vi "Neocera21 Set T.vi"(5 "Channel":i16=1, 6 "Ramp rate, K/min":dbl=1.0, 8 "error in (no error)":errorcluster, 9 "Approach":T1, 10 "Set T":dbl=1.0, 11 "VISA Resource Name":refnum<visa-resource-name>) -> (0 "error out":errorcluster, 3 "VISA Resource Name Out":refnum<visa-resource-name>)   [LabVIEW 2021]
uses:
  Temperature Controller/Controls/Set Point Aproach.ctl
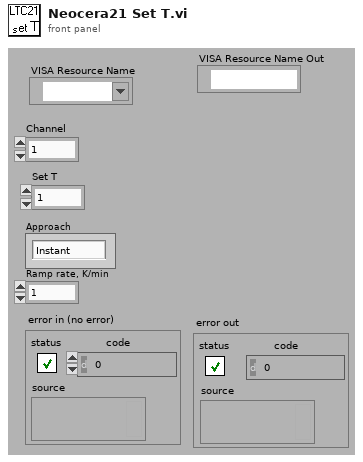
[diagram p1: front panel]
types:
  T1 = typedef "Set Point Aproach.ctl" = enum16{"Instant", "Ramp"}
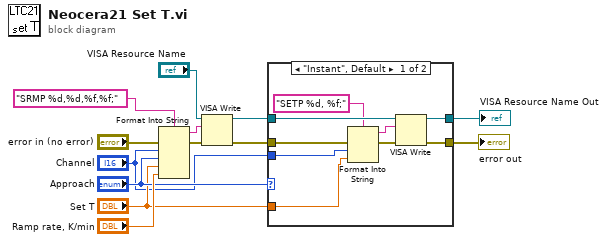
[diagram p0: block diagram]
diagram:
  n1 = Format Into String(format string="SRMP %d,%d,%f,%f;" ("data string"), error in="error in (no error)", "Channel", "Approach", "Set T", "Ramp rate, K/min") -> (resulting string=w10:string, error out=w11:errorcluster)  [unwired: 1 in]
  n2 = VISA Write(VISA resource name="VISA Resource Name", write buffer=w10, error in (no error)=w11) -> (VISA resource name out=w4:refnum<visa-resource-name>, error out=w6:errorcluster)  [unwired: 1 out]
  n3 = case shown="\"Instant\", Default" "Approach" {
    tunnel: w6 -> [w22 w24]
    tunnel: [w21 w24] -> w5
    tunnel: w4 -> [w20 w23]
    tunnel: [w19 w23] -> w3
    tunnel: "Set T" -> [w15 _]
    tunnel: "Channel" -> [w14 _]
    frame "Instant", Default {
      n4 = Format Into String(format string="SETP %d, %f;", error in=w22, w14, w15) -> (resulting string=w16:string, error out=w18:errorcluster)  [unwired: 1 in]
      n5 = VISA Write(VISA resource name=w20, write buffer=w16, error in (no error)=w18) -> (VISA resource name out=w19:refnum<visa-resource-name>, error out=w21:errorcluster)  [unwired: 1 out]
    }
    frame "Ramp" {
    }
  }
  "error out" <- w5
  "VISA Resource Name Out" <- w3
